vi "get_xml_zoom.vi"(8 "error in (no error)":errorcluster, 10 "description XML string in":string, 11 "TrajectoryMH100122AODRAPS in":refnum<class "TrajectoryMH100122AODRAPS.lvclass">) -> (0 "error out":errorcluster, 2 "string out":string, 3 "TrajectoryMH100122AODRAPS out":refnum<class "TrajectoryMH100122AODRAPS.lvclass">)   [LabVIEW 2010]
uses:
  TrajectoryMH100122AODRAPS.lvclass
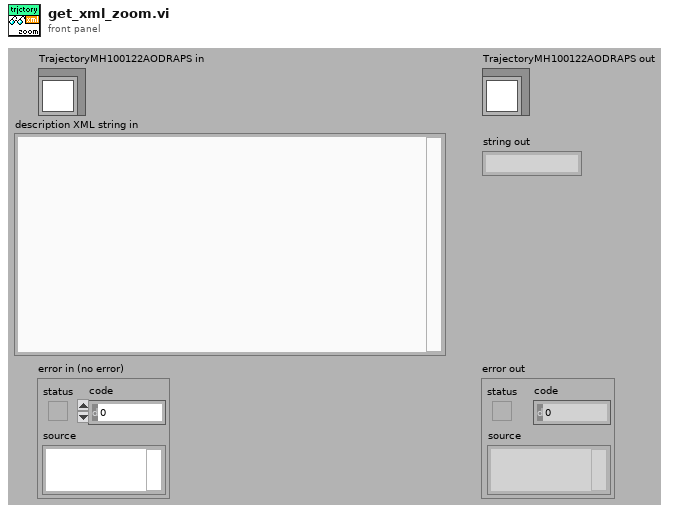
[diagram p1: front panel]
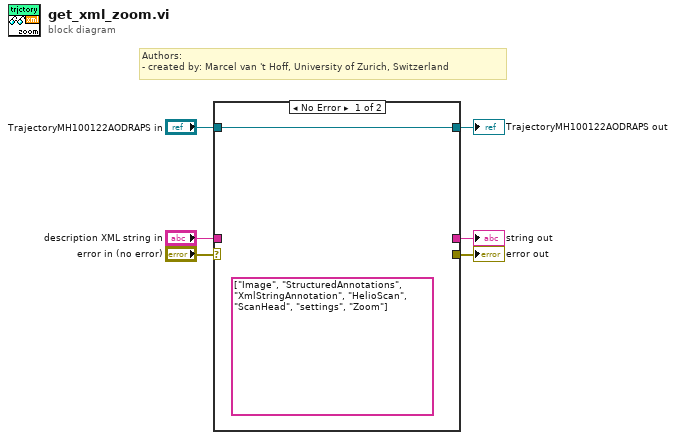
[diagram p0: block diagram]
diagram:
  # "Authors: \n- created by: Marcel van 't Hoff, University of Zurich, Switzerland"
  n1 = case shown="No Error" "error in (no error)" {
    selector: "error in (no error)" -> [w10 w14]
    tunnel: [w9 w14] -> w5
    tunnel: [w12 w13] -> w3
    tunnel: "TrajectoryMH100122AODRAPS in" -> [w12 w13]
    tunnel: "description XML string in" -> [w11 _]
    tunnel: [w8 _] -> w1
    frame No Error {
      w7 = string[] ["Image", "StructuredAnnotations", "XmlStringAnnotation", "HelioScan", "ScanHead", "settings", "Zoom"] ("key chain")
    }
    frame Error {
    }
  }
  "error out" <- w5
  "TrajectoryMH100122AODRAPS out" <- w3
  "string out" <- w1
